vi "Integer2String.vi"(7 "integer":i32) -> (8 "String":string)   [LabVIEW 2022 SP3]
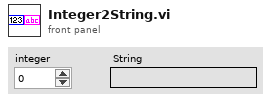
[diagram p1: front panel]
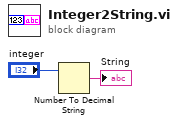
[diagram p0: block diagram]
diagram:
  n1 = Number To Decimal String(number="integer") -> (decimal integer string=→"String":string)  [unwired: 1 in]
